vi "FPGA uint 32 delta Time.vi"() -> (0 "dt":u32)   [LabVIEW 2010]
doc: "Returns the time difference since this was last run. First call returns zero. Unknown behavior in u32 clock overflow case is likely wraparound-> negative large wraps to positive small-> conveniently accurate dt.\nMeasures in milliseconds (ms)"
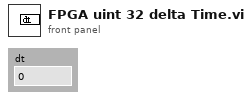
[diagram p1: front panel]
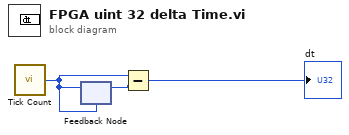
[diagram p0: block diagram]
diagram:
  n1 = call "Tick Count"() -> ("Tick Count(mSec)"=w1:u32)
  n2 = feedback-in #1(w1) -> ()
  n3 = feedback #1(w1) -> (w2:u32)
  n4 = Subtract(x=w1, y=w2) -> (x-y=→"dt":u32)
